vi "Run.vi"(8 "error in (no error)":errorcluster, 9 "s on last turn":dbl, 10 "Maze (0: Empty, -1: Enemy. >0: Teammate":i32[][](array[numeric]), 11 "Expand in":refnum<class "Hesitant Wolf.lvclass">) -> (0 "error out":errorcluster, 1 "Direction":T1, 2 "Action":T2, 3 "Expand out":refnum<class "Hesitant Wolf.lvclass">, 4 "Replicated":refnum<class "Square.lvclass">)   [LabVIEW 2014, in "Hesitant Wolf.lvclass"]
uses:
  Hesitant Wolf.lvclass
  SquareBattle Arena/Action Enum.ctl
  SquareBattle Arena/Direction Enum.ctl
  Square.lvclass
  Hesitant Wolf.lvclass/Hesitant Wolf.ctl
  SquareBattle Arena/SquareBattle Arena.lvclass
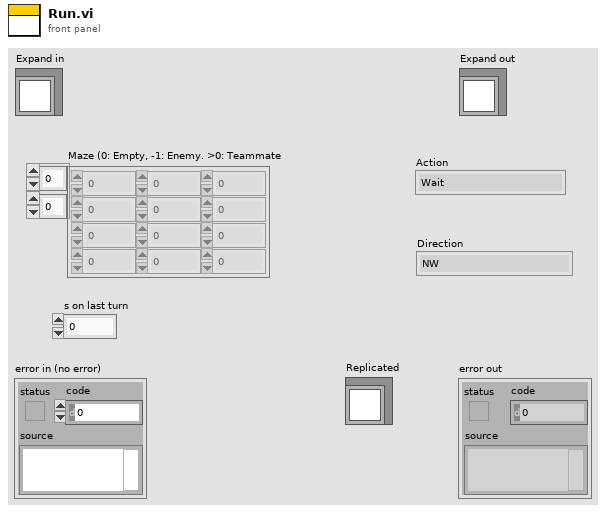
[diagram p1: front panel]
types:
  T1 = typedef "SquareBattle Arena.lvlib/SquareBattle Arena.lvclass/Direction Enum.ctl" = enum16{"NW", "N", "NE", "E", "SE", "S", "SW", "W"}
  T2 = typedef "SquareBattle Arena.lvlib/SquareBattle Arena.lvclass/Action Enum.ctl" = enum16{"Wait", "Move", "Attack", "Replicate"}
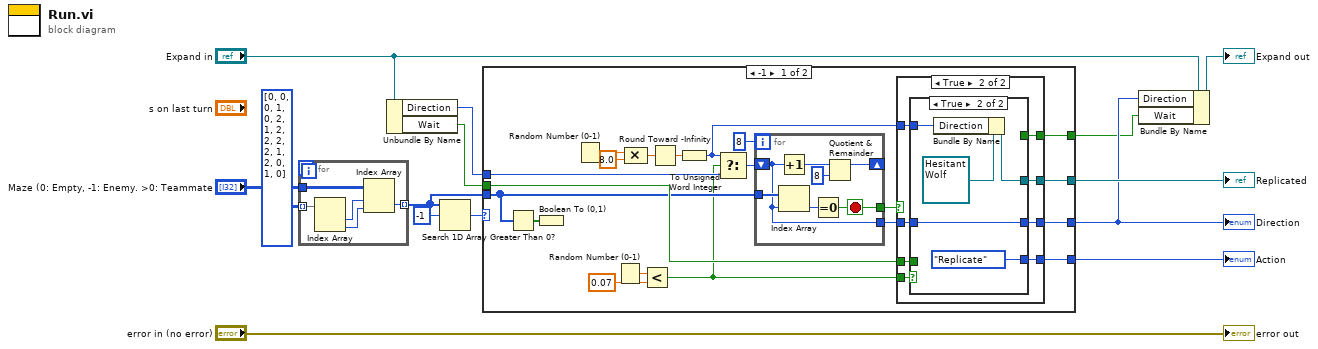
[diagram p0: block diagram]
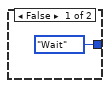
[diagram p2: hidden frame]
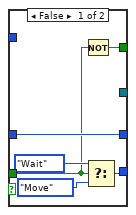
[diagram p3: hidden frame]
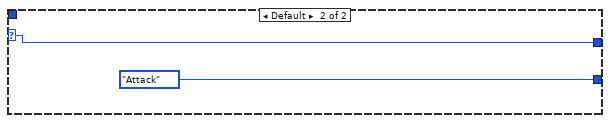
[diagram p4: hidden frame]
diagram:
  n1 = for {
    tunnel: "Maze (0: Empty, -1: Enemy. >0: Teammate" -> [w19]
    tunnel: i32[][] [[0, 0], [0, 1], [0, 2], [1, 2], [2, 2], [2, 1], [2, 0], [1, 0]] -> [w18] mode=indexing
    tunnel: [w15] -> w9 mode=indexing
    n2 = Index Array(array=w18) -> (element #1=w17:i32, element #2=w16:i32)  [unwired: 2 in]
    n3 = Index Array(array=w19, index (row)=w17, index (col)=w16) -> (element=w15:i32)
  }
  n4 = Unbundle By Name("Expand in") -> ("Direction"=w3:T1, "Wait"=w2:bool)
  n5 = Search 1D Array(1D array=w9, element=-1) -> (index of element=w10:i32)  [unwired: 1 in]
  n6 = case shown="-1" w10 {
    selector: w10 -> [_ w67]
    tunnel: [w38 w67] -> w6
    tunnel: [w39 Action_Enum."Attack" ("Action")] -> w7
    tunnel: w9 -> [w22 _]
    tunnel: [w37 _] -> w8
    tunnel: w3 -> [w26 _]
    tunnel: w2 -> [w24 _]
    tunnel: [w23 _] -> w1
    frame -1 {
      n7 = Greater Than 0?(x=w22) -> (x > 0?=w20:bool[])
      n8 = Boolean To (0,1)(Boolean=w20) -> ()  [unwired: 1 out]
      n9 = Random Number (0-1)() -> (number: 0 to 1=w33:dbl)
      n10 = Random Number (0-1)() -> (number: 0 to 1=w35:dbl)
      n11 = Compound Arithmetic op=MULTIPLY(w33, 8.0 ("value")) -> (w31:dbl)
      n12 = Less?(x=w35, y=0.07) -> (x < y?=w21:bool)
      n13 = Round Toward -Infinity(1:w31) -> (0:w30:dbl)
      n14 = To Unsigned Word Integer(number=w30) -> (unsigned 16bit integer=w25:u16)
      n15 = Select(t=w25, s=w21, f=w26) -> (s? t:f=w27:u16)
      n16 = for {
        N: 8 -> [_]
        tunnel: w22 -> [w66]
        shift-right: [w62] -> _
        shift-left: w27 -> [w61]
        tunnel: [w61] -> w29
        tunnel: [w60] -> w28
        stop <- w60 stop-if-true
        n17 = Increment(x=w61) -> (x+1=w64:i32)
        n18 = Index Array(array=w66, index=w61) -> (element=w65:i32)
        n19 = Equal To 0?(x=w65) -> (x = 0?=w60:bool)
        n20 = Quotient & Remainder(x=w64, y=8) -> (x-y*floor(x/y)=w62:i32)  [unwired: 1 out]
      }
      n21 = case shown="True" w28 {
        tunnel: [Action_Enum."Wait" ("y") w48] -> w39
        tunnel: [_ w47] -> w38
        tunnel: [_ w46] -> w37
        tunnel: w21 -> [_ w45]
        tunnel: w29 -> [_ w44]
        tunnel: w25 -> [_ w43]
        tunnel: w24 -> [_ w42]
        tunnel: [_ w41] -> w23
        frame False {
        }
        frame True {
          n22 = case shown="True" w45 {
            tunnel: [w53 Action_Enum."Replicate" ("y")] -> w48
            tunnel: [w54 w58] -> w47
            tunnel: [_ w55] -> w46
            tunnel: w44 -> [w54 w58]
            tunnel: w43 -> [_ w56]
            tunnel: w42 -> [w50 _]
            tunnel: [w49 _] -> w41
            frame False {
              n23 = Not(x=w50) -> (.not. x?=w49:bool)
              n24 = Select(t=Action_Enum."Wait", s=w50, f=Action_Enum."Move" ("y")) -> (s? t:f=w53:T2)
            }
            frame True {
              n25 = Bundle By Name(cluster=refnum<class "Hesitant Wolf.lvclass"> refnum ("Lone Wolf.lvclass"), "Direction"=w56) -> (w55:refnum<class "Hesitant Wolf.lvclass">)
            }
          }
        }
      }
    }
    frame Default {
    }
  }
  "Action" <- w7
  "Direction" <- w6
  "Replicated" <- w8
  n26 = Bundle By Name(cluster="Expand in", "Direction"=w6, "Wait"=w1) -> (→"Expand out":refnum<class "Hesitant Wolf.lvclass">)
  "error out" <- "error in (no error)"
